vi "Limit check (load).vi"(8 "error in (no error)":errorcluster, 11 "Load":dbl) -> (0 "error out":errorcluster, 3 "Limit?":bool)   [LabVIEW 2016]
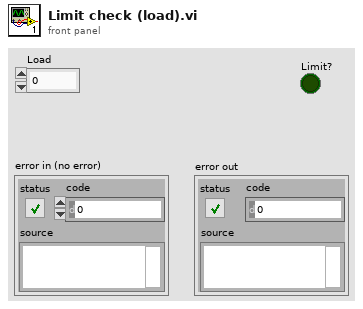
[diagram p1: front panel]
types:
  T1 = typedef "Test settings.ctl" = cluster{"Speed (mm/s)":dbl, "Position limit":bool, "Position limit (mm)":dbl, "Load limit":bool, "Load limit (N)":dbl, "No. of repeats":u16, "Test identifier":string, "Time wait":bool, "Wait time (s)":dbl, "Trigger wait":bool, "Send trigger":bool, "Test notes":string, "Snap intervals":bool, "Time interval (s)":dbl}
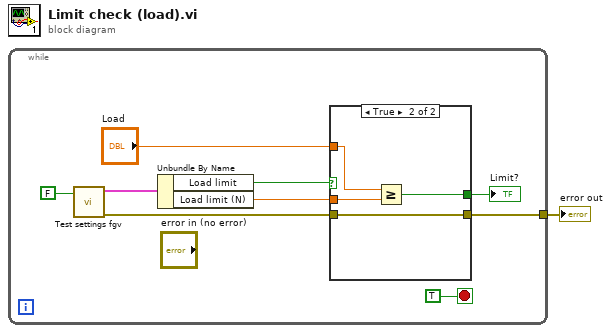
[diagram p0: block diagram]
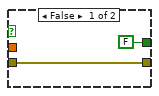
[diagram p2: hidden frame]
diagram:
  n1 = while {
    tunnel: [w2] -> w1
    stop <- TRUE stop-if-true
    n2 = call "Test settings fgv.vi"("Set?"=FALSE) -> ("error out"=w7:errorcluster, "Test settings out"=w9:T1)  [unwired: 8 in, 1 out]
    n3 = Unbundle By Name(w9) -> ("Load limit"=w6:bool, "Load limit (N)"=w5:dbl)
    n4 = case shown="True" w6 {
      tunnel: w5 -> [_ w15]
      tunnel: w7 -> [w12 w13]
      tunnel: "Load" -> [_ w16]
      tunnel: [FALSE w14] -> w3
      tunnel: [w12 w13] -> w2
      frame False {
      }
      frame True {
        n5 = Greater Or Equal?(x=w16, y=w15) -> (x >= y?=w14:bool)
      }
    }
    "Limit?" <- w3
  }
  "error out" <- w1
